vi "Post-Build Custom Action.vi"(10 "Variant":variant) -> (0 "error out":errorcluster)   [LabVIEW 2024]
uses:
  <vilib>/Utility/config.llb/Write Key (String).vi
  <vilib>/Utility/config.llb/NI_LVConfig.lvlib
panel:
  # "Connector Pane"
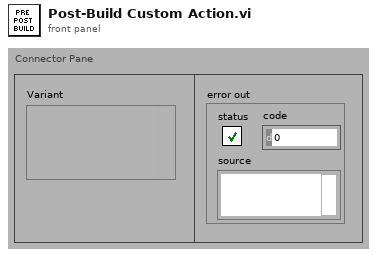
[diagram p1: front panel]
types:
  T1 = typedef "NI_LVConfig.lvlib/Config Data RefNum.ctl" = refnum<k1>
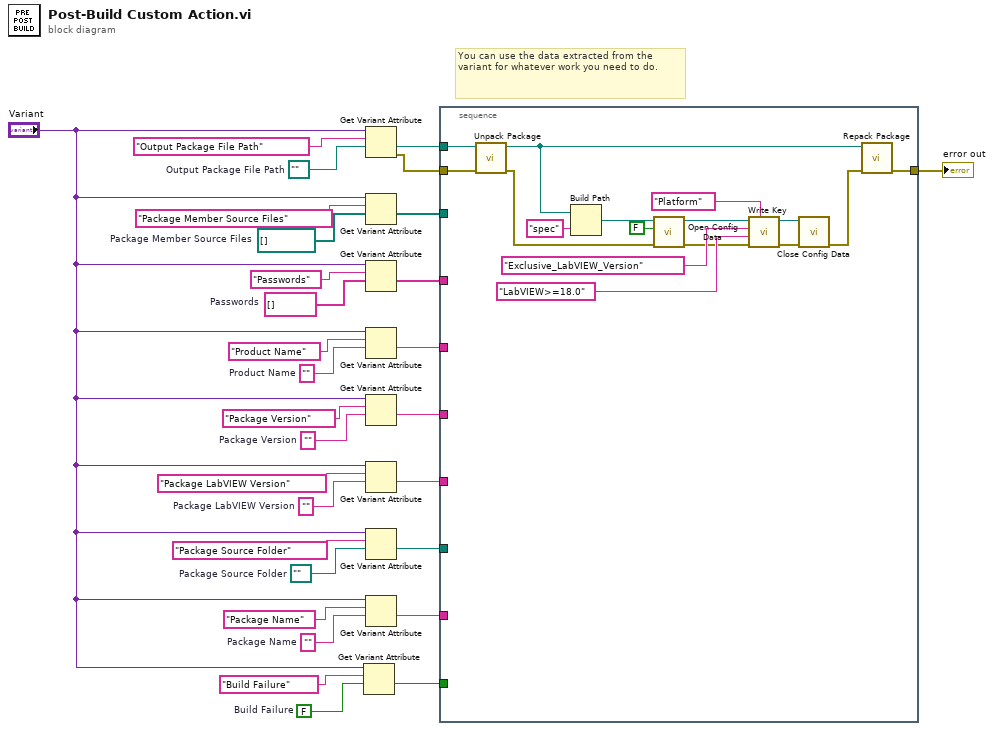
[diagram p0: block diagram]
diagram:
  w5 = FALSE  # Build Failure
  w15 = path ""  # Package Source Folder
  w16 = ""  # Package Name
  w19 = ""  # Package LabVIEW Version
  w21 = ""  # Package Version
  w23 = ""  # Product Name
  w25 = string[] []  # Passwords
  w27 = path[] []  # Package Member Source Files
  w29 = path ""  # Output Package File Path
  # "You can use the data extracted from the variant for whatever work you need to do."
  n1 = Get Variant Attribute(Variant="Variant", name="Build Failure", default value (empty Variant)=w5) -> (value=w3:bool)  [unwired: 1 in, 3 out]
  n2 = Get Variant Attribute(Variant="Variant", name="Output Package File Path", default value (empty Variant)=w29) -> (value=w14:path, error out=w1:errorcluster)  [unwired: 1 in, 2 out]
  n3 = Get Variant Attribute(Variant="Variant", name="Package Member Source Files", default value (empty Variant)=w27) -> (value=w13:path[])  [unwired: 1 in, 3 out]
  n4 = Get Variant Attribute(Variant="Variant", name="Passwords", default value (empty Variant)=w25) -> (value=w12:string[])  [unwired: 1 in, 3 out]
  n5 = Get Variant Attribute(Variant="Variant", name="Product Name", default value (empty Variant)=w23) -> (value=w11:string)  [unwired: 1 in, 3 out]
  n6 = Get Variant Attribute(Variant="Variant", name="Package Version", default value (empty Variant)=w21) -> (value=w10:string)  [unwired: 1 in, 3 out]
  n7 = Get Variant Attribute(Variant="Variant", name="Package LabVIEW Version", default value (empty Variant)=w19) -> (value=w9:string)  [unwired: 1 in, 3 out]
  n8 = Get Variant Attribute(Variant="Variant", name="Package Source Folder", default value (empty Variant)=w15) -> (value=w8:path)  [unwired: 1 in, 3 out]
  n9 = Get Variant Attribute(Variant="Variant", name="Package Name", default value (empty Variant)=w16) -> (value=w7:string)  [unwired: 1 in, 3 out]
  n10 = stacked-sequence {
    tunnel: w14 -> [w46]
    tunnel: w13 -> [_]
    tunnel: w12 -> [_]
    tunnel: w11 -> [_]
    tunnel: w10 -> [_]
    tunnel: w9 -> [_]
    tunnel: w8 -> [_]
    tunnel: w7 -> [_]
    tunnel: w3 -> [_]
    tunnel: [w33] -> w2
    tunnel: w1 -> [w31]
    frame #0 {
      n11 = call "Unpack Package.vi"("error in (no error)"=w31, "Package File"=w46) -> ("error out"=w32:errorcluster, "Unpacked Package Directory"=w35:path)  [unwired: 7 in, 1 out]
      n12 = Build Path(base path=w35, name or relative path="spec") -> (appended path=w44:path)
      n13 = call <vilib>:"Open Config Data.vi"("error in (no error)"=w32, "create file if necessary (T)"=FALSE, "configuration file path"=w44) -> ("error out"=w38:errorcluster, "refnum"=w42:T1)  [unwired: 6 in, 1 out]
      n14 = call-poly <vilib>:"Write Key.vi"("section"="Platform", "error in (no error)"=w38, "value"="LabVIEW>=18.0", "key"="Exclusive_LabVIEW_Version", "refnum"=w42) -> ("error out"=w36:errorcluster, "refnum out"=w37:T1)  [unwired: 4 in, 1 out]
      n15 = call <vilib>:"Close Config Data.vi"("error in (no error)"=w36, "refnum"=w37) -> ("error out"=w34:errorcluster)  [unwired: 8 in, 1 out]
      n16 = call "Repack Package.vi"("error in (no error)"=w34, "Directory to repack"=w35) -> ("error out"=w33:errorcluster)  [unwired: 9 in]
    }
  }
  "error out" <- w2
